vi "Place_Middle_Gear_Auto.vi"(0 "Encoder_In":dbl, 5 "Yaw_In":dbl, 7 "Place_Finished?":bool, 9 "Reverse_Drive_Speed":dbl=-0.5 format="%#_13g", 11 "Reverse_Drive_Distance":dbl=84.0, 12 "Start?":bool) -> (4 "Drive_PID_Enable":bool, 6 "Place_Gear?":bool, 8 "Current_State":enum16{"Idle", "Drive", "Place_Gear"}(ring), 10 "Desired_Yaw":dbl)   [LabVIEW 2016]
panel:
  out "Drive_Speed":dbl
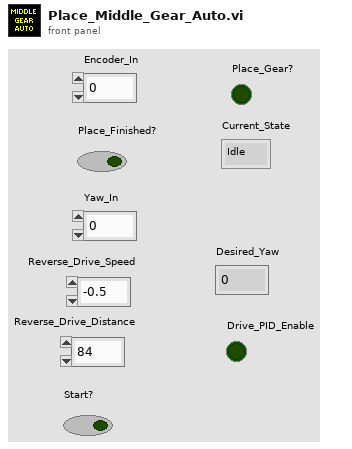
[diagram p1: front panel]
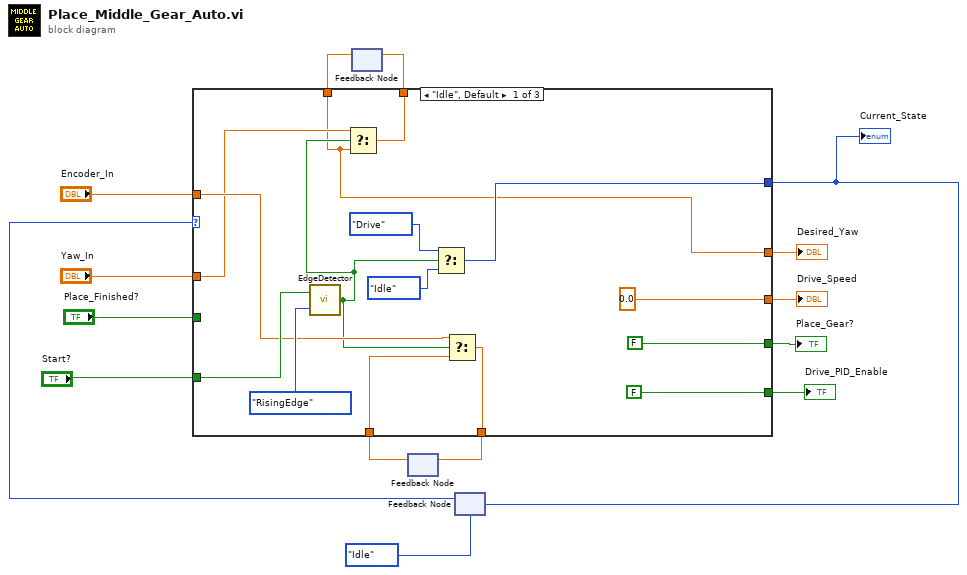
[diagram p0: block diagram]
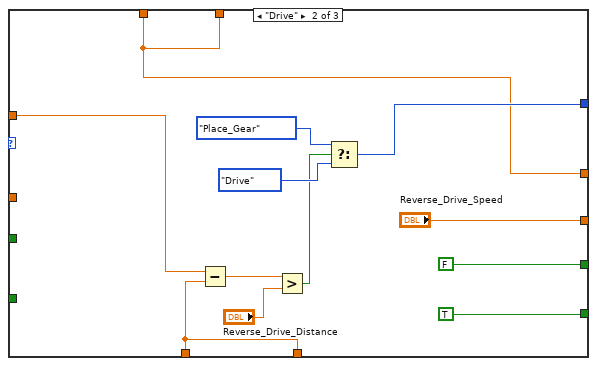
[diagram p2: hidden frame]
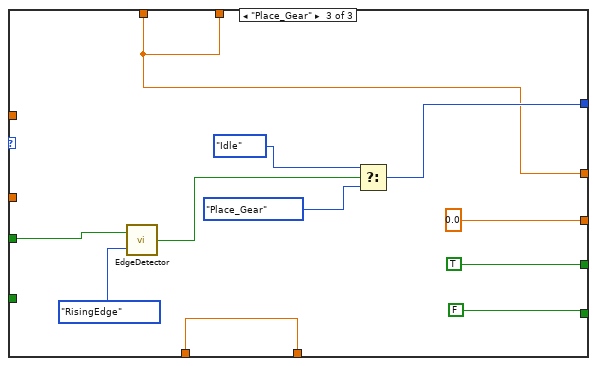
[diagram p3: hidden frame]
diagram:
  n1 = feedback #1() -> (w4:dbl)  [unwired: 1 in]
  n2 = feedback #2() -> (w6:dbl)  [unwired: 1 in]
  n3 = feedback #3(enum16{"Idle", "Drive", "Place_Gear"}."Idle") -> (w13:enum16{"Idle", "Drive", "Place_Gear"})
  n4 = case shown="\"Idle\", Default" w13 {
    tunnel: "Encoder_In" -> [w23 w38 _]
    tunnel: "Start?" -> [w29 _ _]
    tunnel: [w26 w41 w51] -> w12
    tunnel: [FALSE FALSE TRUE] -> w11
    tunnel: [0.0 ("Drive_Speed") "Reverse_Drive_Speed" 0.0 ("Drive_Speed")] -> w10
    tunnel: "Place_Finished?" -> [_ _ w53]
    tunnel: "Yaw_In" -> [w20 _ _]
    tunnel: [w22 w33 w45] -> w7
    tunnel: w6 -> [w21 w33 w45]
    tunnel: [w18 w32 w44] -> w5
    tunnel: w4 -> [w17 w32 w44]
    tunnel: [w17 w32 w44] -> w3
    tunnel: [FALSE TRUE FALSE] -> w2
    frame "Idle", Default {
      n5 = call "EdgeDetector.vi"("DetectorType"=enum16{"RisingEdge", "FallingEdge", "Both"}."RisingEdge", "Input"=w29) -> ("Edge"=w19:bool)
      n6 = Select(t=w20, s=w19, f=w17) -> (s? t:f=w18:dbl)
      n7 = Select(t=enum16{"Idle", "Drive", "Place_Gear"}."Drive", s=w19, f=enum16{"Idle", "Drive", "Place_Gear"}."Idle") -> (s? t:f=w26:enum16{"Idle", "Drive", "Place_Gear"})
      n8 = Select(t=w23, s=w19, f=w21) -> (s? t:f=w22:dbl)
    }
    frame "Drive" {
      n9 = Subtract(x=w38, y=w33) -> (x-y=w37:dbl)
      n10 = Greater?(x=w37, y="Reverse_Drive_Distance") -> (0:w34:bool)
      n11 = Select(t=enum16{"Idle", "Drive", "Place_Gear"}."Place_Gear", s=w34, f=enum16{"Idle", "Drive", "Place_Gear"}."Drive") -> (s? t:f=w41:enum16{"Idle", "Drive", "Place_Gear"})
    }
    frame "Place_Gear" {
      n12 = call "EdgeDetector.vi"("DetectorType"=enum16{"RisingEdge", "FallingEdge", "Both"}."RisingEdge", "Input"=w53) -> ("Edge"=w49:bool)
      n13 = Select(t=enum16{"Idle", "Drive", "Place_Gear"}."Idle", s=w49, f=enum16{"Idle", "Drive", "Place_Gear"}."Place_Gear") -> (s? t:f=w51:enum16{"Idle", "Drive", "Place_Gear"})
    }
  }
  "Place_Gear?" <- w11
  "Current_State" <- w12
  "Drive_Speed" <- w10
  "Desired_Yaw" <- w3
  "Drive_PID_Enable" <- w2
  n14 = feedback-in #1(w5) -> ()
  n15 = feedback-in #2(w7) -> ()
  n16 = feedback-in #3(w12) -> ()
